vi "saveInstrumentsScripts.vi"(8 "error in (no error)":errorcluster, 11 "ScriptListCompiler in":refnum<class "ScriptListCompiler.lvclass">) -> (0 "error out":errorcluster, 3 "ScriptListCompiler out":refnum<class "ScriptListCompiler.lvclass">)   [LabVIEW 2009, in "Compiler.lvlib" / "ScriptListCompiler.lvclass"]
uses:
  ScriptListCompiler.lvclass
  ScriptListCompiler.lvclass/ScriptListCompiler.ctl
  Filing/FileNeologist/FileNeologist.lvclass
  DatabaseHelpers/Database Objects/device/device.lvclass
  DatabaseHelpers/Database Objects/DeviceArray/DeviceArray.lvclass
  Filing.lvlib
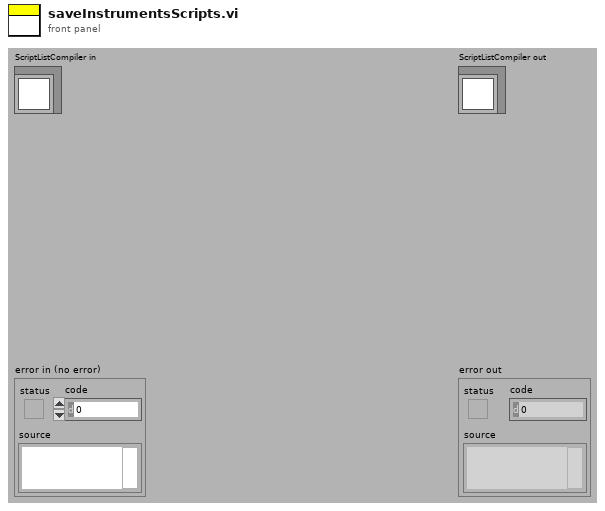
[diagram p1: front panel]
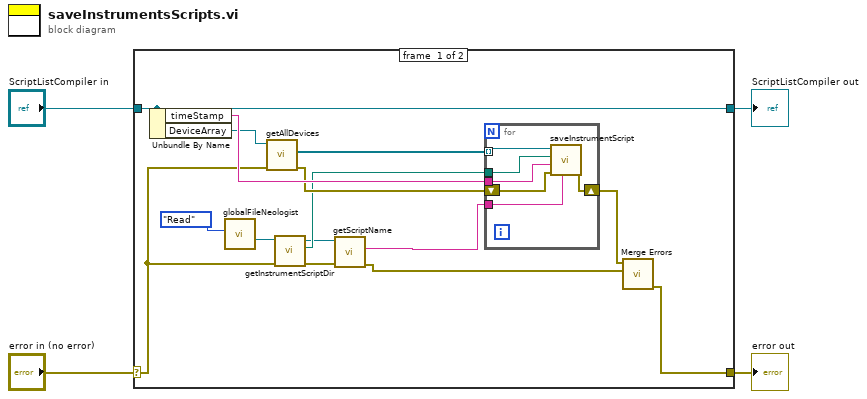
[diagram p0: block diagram]
diagram:
  n1 = case shown="No Error" "error in (no error)" {
    selector: "error in (no error)" -> [w11 w27]
    tunnel: [w9 w27] -> w3
    tunnel: [w19 w26] -> w1
    tunnel: "ScriptListCompiler in" -> [w19 w26]
    frame #0 {
      n2 = Unbundle By Name(w19) -> ("timeStamp"=w17:string, "DeviceArray"=w15:refnum<class "DeviceArray.lvclass">)
      n3 = call "globalFileNeologist.vi"("Action"=enum16{"Write", "Read"}."Read") -> ("FileNeologist out"=w13:refnum<class "FileNeologist.lvclass">)  [unwired: 10 in]
      n4 = call "getAllDevices.vi"("error in (no error)"=w11, "DeviceArray.lvclass in"=w15) -> ("error out"=w16:errorcluster, "deviceArray"=w18:refnum<class "device.lvclass">[])  [unwired: 7 in, 1 out]
      n5 = call "getInstrumentScriptDir.vi"("error in (no error)"=w11, "FileNeologist in"=w13) -> ("error out"=w8:errorcluster, "instrumentScript dir"=w12:path, "FileNeologist out"=w7:refnum<class "FileNeologist.lvclass">)  [unwired: 7 in]
      n6 = call-dynamic "getScriptName.vi"("error in (no error)"=w8, "FileNeologist.lvclass in"=w7) -> ("error out"=w5:errorcluster, "scriptName"=w6:string)  [unwired: 7 in, 1 out]
      n7 = for {
        tunnel: w18 -> [w25] mode=indexing
        tunnel: w12 -> [w24]
        tunnel: w17 -> [w23]
        shift-right: [w22] -> w10
        shift-left: w16 -> [w21]
        tunnel: w6 -> [w20]
        n8 = call "saveInstrumentScript.vi"("scriptName"=w20, "error in (no error)"=w21, "timeStamp"=w23, "folderPath"=w24, "device in"=w25) -> ("error out"=w22:errorcluster)  [unwired: 5 in, 1 out]
      }
      n9 = call <vilib>:"Merge Errors.vi"("error in 2 (no error)"=w5, "error in 1 (no error)"=w10) -> ("error out"=w9:errorcluster)  [unwired: 5 in]
    }
    frame #1 {
    }
  }
  "error out" <- w3
  "ScriptListCompiler out" <- w1
